vi "AuMT8852B EDR Fail Register Query.vi"(8 "error in (no error)":errorcluster, 11 "VISA session":refnum<visa-resource-name>) -> (0 "error out":errorcluster, 2 "error code":i32, 3 "VISA session out":refnum<visa-resource-name>, 4 "Flags":T1 {"Max Input Power" items=["Max input power passed", "Max input power failed"]; "BER Floor Sensitivity" items=["BER floor sensitivity passed", "BER floor sensitivity failed"]; "Sensitivity" items=["Sensitivity passed", "Sensitivity failed"]; "Differential Phase Encoding" items=["Differential phase passed", "Differential phase failed"]; "Carrier frequency & Mod" items=["Carrier frequency & mod passed", "Carrier frequency & mod failed"]; "Relative Transmit Power" items=["Relative transmit power passed", "Relative transmit power failed"]}, 6 "Value":i32)   [LabVIEW 2017]
doc: "Anritsu MT8852B Bluetooth Tester\n\nReturns an integer containg one bit for each Bluetooth test. Each bit is 0 if the test passed and 1 if the test failed.\n\nBit 5 (most significant bit) - Maximum input power test.\nBit 4 - BER floor sensitivity test.\nBit 3 - Sensitivity test.\nBit 2 - Differential phase encoding test.\nBit 1 - Carrier stability and modulation accuracy test.\nBit 0 (least significant bit) - Relative transmit power test.\n\nOUTPUTS\nFlags - status of each test in the register.\nValue - integer value (0-255) of the register."
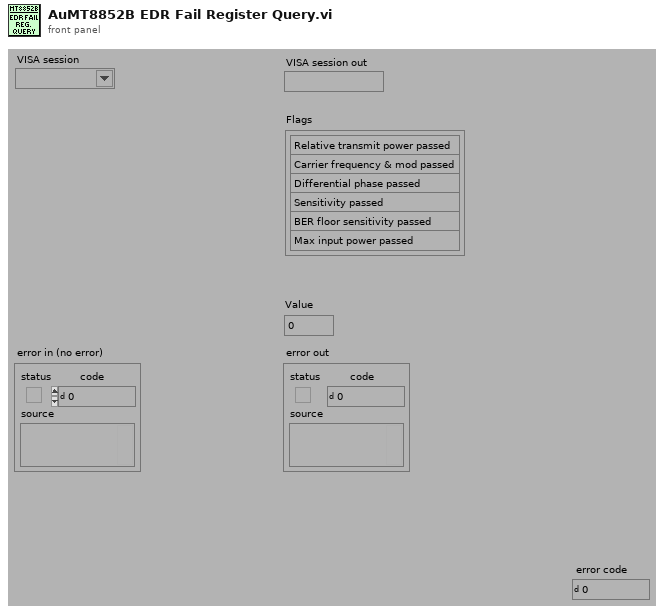
[diagram p1: front panel]
types:
  T1 = cluster{"Relative Transmit Power":u16, "Carrier frequency & Mod":u16, "Differential Phase Encoding":u16, "Sensitivity":u16, "BER Floor Sensitivity":u16, "Max Input Power":u16}
  T2 = enum16{"Simulate", "Range check", "Cache", "Query instrument status"}
  T3 = cluster{"[0]":i16, "[1]":i16, "[2]":i16, "[3]":i16, "[4]":i16, "[5]":i16}
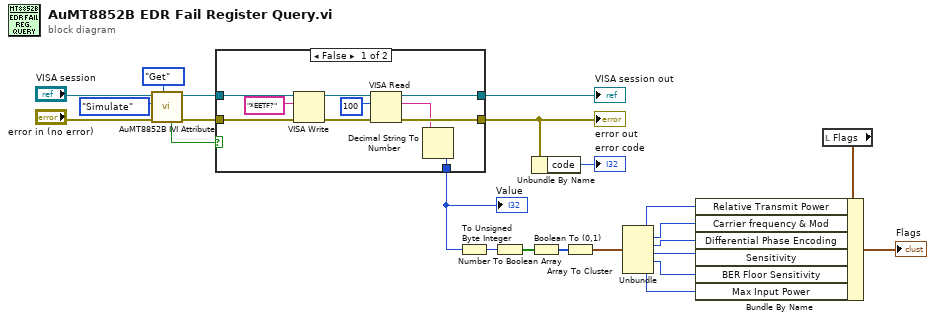
[diagram p0: block diagram]
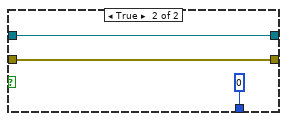
[diagram p2: hidden frame]
diagram:
  n1 = call <instrlib>:"AuMT8852B IVI Attribute.vi"("Set/Get (Set)"=enum16{"Set", "Get"}."Get", "error in (no error)"="error in (no error)", "Flag (Simulate)"=T2."Simulate", "VISA session"="VISA session") -> ("error out"=w19:errorcluster, "VISA session out"=w20:refnum<visa-resource-name>, "Value out"=w16:bool)  [unwired: 5 in]
  n2 = case shown="False" w16 {
    tunnel: [w27 w35] -> w11
    tunnel: [w28 w36] -> w21
    tunnel: w20 -> [w33 w36]
    tunnel: w19 -> [w32 w35]
    tunnel: [w24 0] -> w10
    frame False {
      n3 = VISA Write(VISA resource name=w33, write buffer="*EETF?" ("write buffer (\"\")"), error in (no error)=w32) -> (VISA resource name out=w30:refnum<visa-resource-name>, error out=w29:errorcluster)  [unwired: 1 out]
      n4 = VISA Read(VISA resource name=w30, byte count=u32 100 ("byte count (0)"), error in (no error)=w29) -> (VISA resource name out=w28:refnum<visa-resource-name>, read buffer=w25:string, error out=w27:errorcluster)  [unwired: 1 out]
      n5 = Decimal String To Number(string=w25) -> (number=w24:i32)  [unwired: 2 in, 1 out]
    }
    frame True {
    }
  }
  "error out" <- w11
  "VISA session out" <- w21
  "Value" <- w10
  n6 = To Unsigned Byte Integer(number=w10) -> (unsigned 8bit integer=w15:u8)
  n7 = Number To Boolean Array(number=w15) -> (Boolean array=w14:bool[])
  n8 = Boolean To (0,1)(Boolean=w14) -> (0, 1=w13:i16[])
  n9 = Unbundle By Name(w11) -> ("code"=→"error code":i32)
  n10 = Array To Cluster(array=w13) -> (cluster=w9:T3)
  n11 = Unbundle(w9) -> ("[0]"=w1:i16, "[1]"=w2:i16, "[2]"=w5:i16, "[3]"=w6:i16, "[4]"=w4:i16, "[5]"=w3:i16)
  n12 = local read "Flags"() -> (w8:T1)
  n13 = Bundle By Name(cluster=w8, "Relative Transmit Power"=w1, "Carrier frequency & Mod"=w2, "Differential Phase Encoding"=w5, "Sensitivity"=w6, "BER Floor Sensitivity"=w4, "Max Input Power"=w3) -> (→"Flags":T1)
